vi "Data acquisition.vi"(0 "Current range":dbl=150.0 min=150.0 max=200.0 step=1.0, 5 "Stop":bool, 7 "Temperature range":dbl=50.0 min=30.0 max=50.0 step=1.0, 11 "Error in":errorcluster) -> (4 "Current indicator":dbl, 8 "Temperature indicator":dbl, 15 "Error out":errorcluster)   [LabVIEW 2020]
doc: "This VI is used to acquire data which is used to generate current and voltage values in a specified range"
uses:
  Typedefs/Data cluster.ctl
  Typedefs/Stop cases.ctl
panel:
  # "Data Acquisition"
  # "OUTPUT"
  # "INPUT"
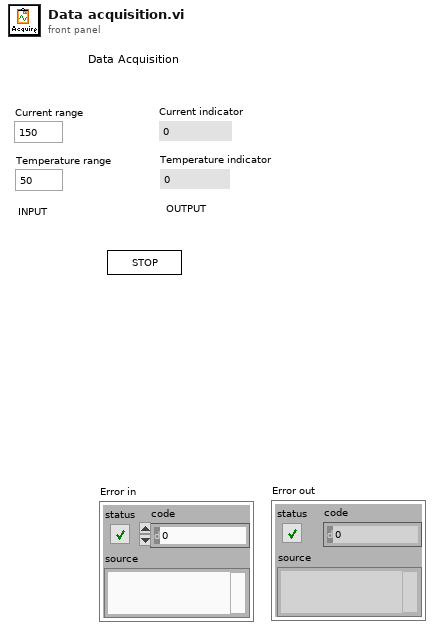
[diagram p1: front panel]
types:
  T1 = typedef "Stop cases.ctl" = enum16{"Initialize", "Write", "Stop"}
  T2 = typedef "Data cluster.ctl" = cluster{"Current":i32, "Temperature":i32}
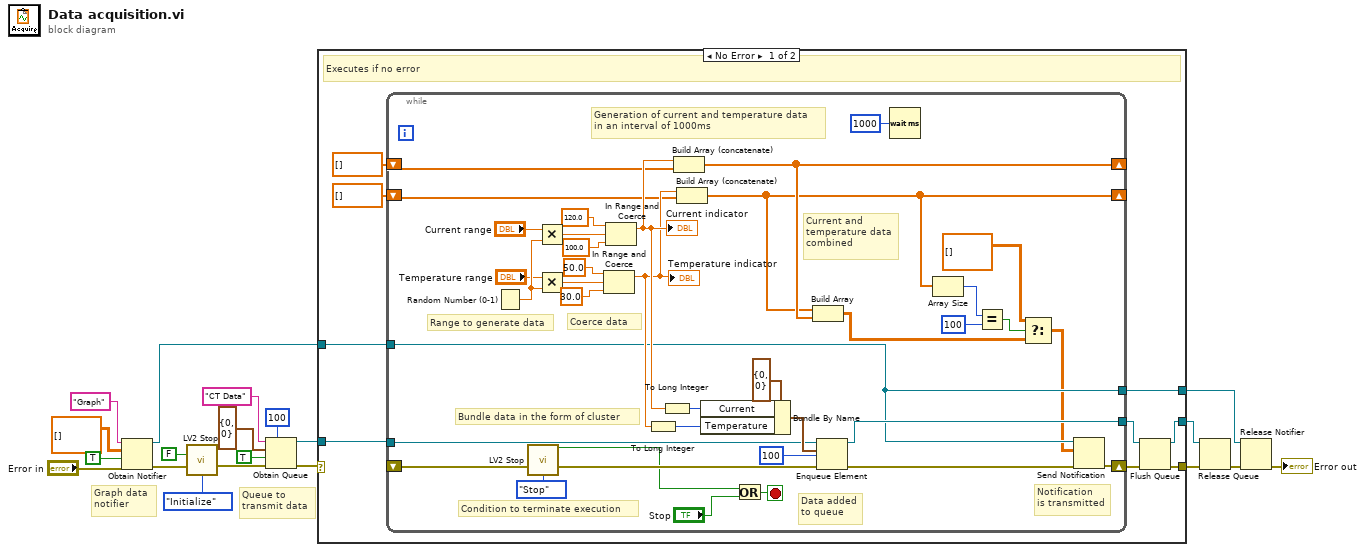
[diagram p0: block diagram]
diagram:
  # "Graph data \nnotifier"
  # "Queue to \ntransmit data"
  n1 = Obtain Notifier(name (unnamed)="Graph", notification data type=dbl[][] [], create if not found? (T)=TRUE, error in (no error)="Error in") -> (notifier out=w2:refnum<notifier>, error out=w15:errorcluster)  [unwired: 1 out]
  n2 = call "LV2 Stop.vi"("Stop"=FALSE, "Error in"=w15, "Operation"=Stop_cases."Initialize") -> ("Error out"=w14:errorcluster)  [unwired: 11 in, 1 out]
  n3 = Obtain Queue(max queue size (-1, unlimited)=100, name (unnamed)="CT Data", element data type=T2 {"Current"=0, "Temperature"=0} ("CT Data"), create if not found? (T)=TRUE, error in (no error)=w14) -> (queue out=w3:refnum<queue>, error out=w4:errorcluster)  [unwired: 1 out]
  n4 = case shown="No Error" w4 {
    selector: w4 -> [_ w70]
    tunnel: [w23 w70] -> w20
    tunnel: [w21 w68] -> w17
    tunnel: [w27 w69] -> w16
    tunnel: w3 -> [w26 w68]
    tunnel: w2 -> [w25 w69]
    frame No Error {
      # "Executes if no error"
      n5 = while {
        shift-right: [w36] -> _
        shift-left: dbl[] [] -> [w40]
        shift-right: [w45] -> w24
        shift-left: _ -> [w58]
        tunnel: w25 -> [w37]
        tunnel: w26 -> [w44]
        shift-right: [w39] -> _
        shift-left: dbl[] [] -> [w42]
        tunnel: [w38] -> w22
        tunnel: [w37] -> w27
        stop <- w54 stop-if-true
        # "Current and\ntemperature data\ncombined"
        # "Notification \nis transmitted"
        # "Data added\nto queue"
        # "Condition to terminate execution"
        # "Bundle data in the form of cluster"
        # "Coerce data"
        # "Range to generate data"
        # "Generation of current and temperature data\nin an interval of 1000ms"
        n6 = Random Number (0-1)() -> (number: 0 to 1=w66:dbl)
        n7 = call "LV2 Stop.vi"("Error in"=w58, "Operation"=Stop_cases."Stop") -> ("Output"=w47:bool, "Error out"=w57:errorcluster)  [unwired: 12 in]
        n8 = Multiply(x="Current range", y=w66) -> (x*y=w51:dbl)
        n9 = Multiply(x="Temperature range", y=w66) -> (x*y=w48:dbl)
        n10 = In Range and Coerce(upper limit=50.0, x=w48, lower limit=30.0) -> (coerced(x)=w41:dbl)  [unwired: 1 out]
        "Temperature indicator" <- w41
        n11 = In Range and Coerce(upper limit=120.0, x=w51, lower limit=100.0) -> (coerced(x)=w43:dbl)  [unwired: 1 out]
        "Current indicator" <- w43
        n12 = To Long Integer(number=w41) -> (32bit integer=w61:i32)
        n13 = To Long Integer(number=w43) -> (32bit integer=w60:i32)
        n14 = Build Array (concatenate)(w43, w42) -> (w39:dbl[])
        n15 = Build Array (concatenate)(w41, w40) -> (w36:dbl[])
        n16 = Bundle By Name(cluster=T2 {"Current"=0, "Temperature"=0} ("CT Data"), "Current"=w60, "Temperature"=w61) -> (w63:T2)
        n17 = Or(x=w47, y="Stop") -> (x .or. y?=w54:bool)
        n18 = Build Array(w36, w39) -> (w31:dbl[][])
        n19 = Enqueue Element(queue=w44, element=w63, timeout in ms (-1)=100, error in (no error)=w57) -> (queue out=w38:refnum<queue>, error out=w46:errorcluster)  [unwired: 1 out]
        n20 = Wait (ms)(milliseconds to wait=u32 1000) -> ()  [unwired: 1 out]
        n21 = Array Size(array=w36) -> (size(s)=w34:i32)
        n22 = Equal?(x=w34, y=100) -> (x = y?=w35:bool)
        n23 = Select(t=dbl[][] [], s=w35, f=w31) -> (s? t:f=w30:dbl[][])
        n24 = Send Notification(notification=w30, notifier=w37, error in (no error)=w46) -> (error out=w45:errorcluster)  [unwired: 1 out]
      }
      n25 = Flush Queue(queue=w22, error in (no error)=w24) -> (queue out=w21:refnum<queue>, error out=w23:errorcluster)  [unwired: 1 out]
    }
    frame Error {
      # "Terminate execution if there is any error"
    }
  }
  n26 = Release Queue(queue=w17, error in (no error)=w20) -> (error out=w19:errorcluster)  [unwired: 1 in, 2 out]
  n27 = Release Notifier(notifier=w16, error in (no error)=w19) -> (error out=→"Error out":errorcluster)  [unwired: 1 in, 2 out]
